vi "2L22_SPOP_estime_facteur_correctif.vi"(1 "Taille de l'échantillon":u32, 2 "Taille population":u32) -> (0 "facteur S":dbl)   [LabVIEW 2010, in "lv_02.lvlib"]
doc: "Ce vi calcule le facteur correctif lors d'un tirage sans remise lorsque la population (pop) est finie de taille N_pop. Quand N devient grand devient n, ce coefficient tends vers 1.\nSi N n'est pas supérieur à 1 alors, le facteur est rendu à 1."
uses:
  lv_02.lvlib
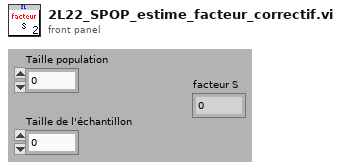
[diagram p1: front panel]
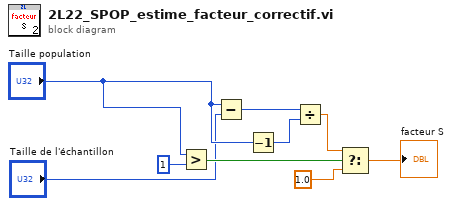
[diagram p0: block diagram]
diagram:
  n1 = Greater?(x="Taille population", y=u32 1) -> (0:w6:bool)
  n2 = Subtract(x="Taille population", y="Taille de l'échantillon") -> (x-y=w2:u32)
  n3 = Decrement(x="Taille population") -> (x-1=w3:u32)
  n4 = Divide(x=w2, y=w3) -> (x/y=w8:dbl)
  n5 = Select(t=w8, s=w6, f=1.0 ("cas faux")) -> (s? t:f=→"facteur S":dbl)
